vi "Distance Sensor-DM.vi"(2 "NXT":T1={"Hardware"="NXT", "Flattened String"=""}, 3 "Input Port":T2 items=["Port 1", "Port 2", "Port 3", "Port 4"]) -> (1 "Output of Distance Sensor":cluster{"Distance Value":ext, "Status":bool}, 4 "NXT dup":T1={"Hardware"="NXT", "Flattened String"=""} caption="NXT")   [LabVIEW 2012]
uses:
  <vilib>/NXT/Subs/LVHSConnector.ctl
  <vilib>/NXT/Block Support/NXT_InputPort.ctl
  <vilib>/NXT/Block Support/HWPage.SensorType.ctl
  <vilib>/NXT/Block Support/HWPage.SensorMode.ctl
panel:
  out "Distance Value":ext
  out "Status (boolean)":bool caption="Success?"
  out "Sensor Type 2":u8(ring) items=["none"=49, "short"=50, "medium"=51, "long"=52, "none"=53]
  out "Sensor Type":u8(ring) items=["GP2D12"=49, "GP2D120"=50, "GP2YA21"=51, "GP2YA02"=52, "CUSTOM"=53]
  # "mindsensors.com\nCopyright (c) 2009 by mindsensors.com\nEmail: info (<at>) mindsensors (<dot>) com\n\nThis program is free software. You can redistribute it and/or modify\nit under the terms of the GNU General Public License as published by\nthe Free Software Foundation; version 3 of the License.\nRead the license at: http://www.gnu.org/licenses/gpl.txt"
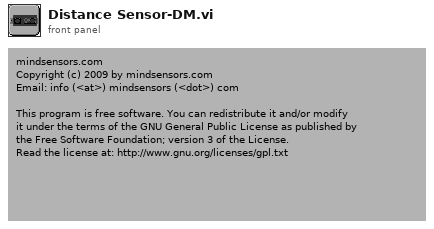
[diagram p1: front panel]
types:
  T1 = typedef "LVHSConnector.ctl" = cluster{"Hardware":string, "Flattened String":string}
  T2 = typedef "NXT_InputPort.ctl" = u8
  T3 = typedef "HWPage.SensorType.ctl" = u8
  T4 = typedef "HWPage.SensorMode.ctl" = u8
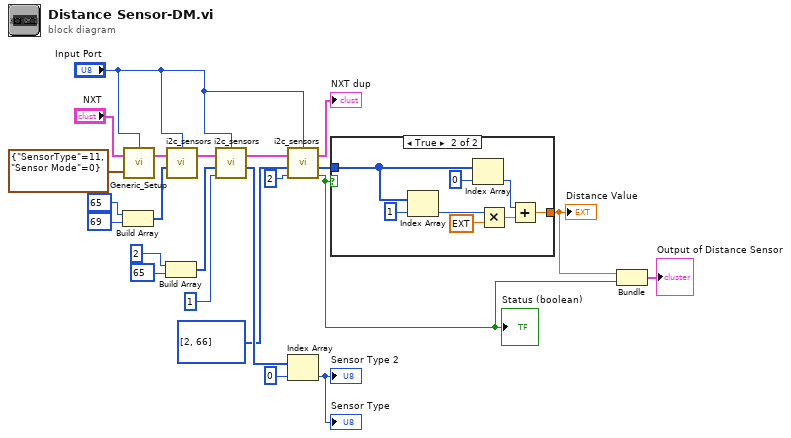
[diagram p0: block diagram]
diagram:
  n1 = Build Array(u8 65 ("Reg Address"), 69) -> (w18:i32[])
  n2 = call <vilib>:"Generic_Setup.vi"("Sensor Setup"=cluster{"SensorType":T3, "Sensor Mode":T4} {"SensorType"=11, "Sensor Mode"=0}, "NXT"="NXT", "Port"="Input Port") -> ("NXT"=w10:T1)  [unwired: 1 out]
  n3 = Build Array(u8 2 ("Device Address"), u8 65 ("Reg Address")) -> (w14:u8[])
  n4 = call <vilib>:"i2c_sensors.vi"("Bytes to Write"=w18, "NXT"=w10, "Port"="Input Port") -> ("NXT"=w21:T1)  [unwired: 2 in, 2 out]
  n5 = call <vilib>:"i2c_sensors.vi"("Return Length"=u8 1 ("bytes to read"), "Bytes to Write"=w14, "NXT"=w21, "Port"="Input Port") -> ("Bytes read"=w13:u8[], "NXT"=w5:T1)  [unwired: 1 in, 1 out]
  n6 = call <vilib>:"i2c_sensors.vi"("Return Length"=u8 2, "Bytes to Write"=u8[] [2, 66] ("Parameters"), "NXT"=w5, "Port"="Input Port") -> ("Success?"=w3:bool, "Bytes read"=w7:u8[], "NXT"=→"NXT dup":T1)  [unwired: 1 in]
  "Status (boolean)" <- w3
  n7 = Index Array(array=w13, index=0) -> (element=→"Sensor Type" →"Sensor Type 2":u8)
  n8 = case shown="True" w3 {
    tunnel: w7 -> [_ w27]
    tunnel: [_ w24] -> w4
    frame False {
    }
    frame True {
      n9 = Index Array(array=w27, index=1) -> (element=w29:u8)
      n10 = Index Array(array=w27, index=0) -> (element=w26:u8)
      n11 = Multiply(x=w29, y=ext 256.0) -> (x*y=w25:ext)
      n12 = Add(x=w26, y=w25) -> (x+y=w24:ext)
    }
  }
  "Distance Value" <- w4
  n13 = Bundle(w4, "Success?"=w3) -> (→"Output of Distance Sensor":cluster{ext, "Success?":bool})  [unwired: 1 in]
